vi "house_model.vi"(0 "T_out":dbl=5.0, 1 "dt":dbl=0.01, 5 "t_0":dbl, 9 "T_room_0":dbl, 14 "heat_level":dbl) -> (3 "heat_loss":dbl, 4 "T_room":dbl, 6 "error_code":dbl, 8 "t":dbl, 10 "T_heater":dbl, 15 "heat_flow":dbl)   [LabVIEW 2014]
panel:
  in  "T_heater_0":dbl
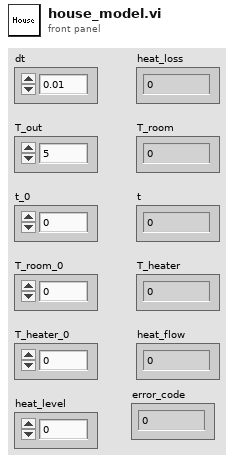
[diagram p1: front panel]
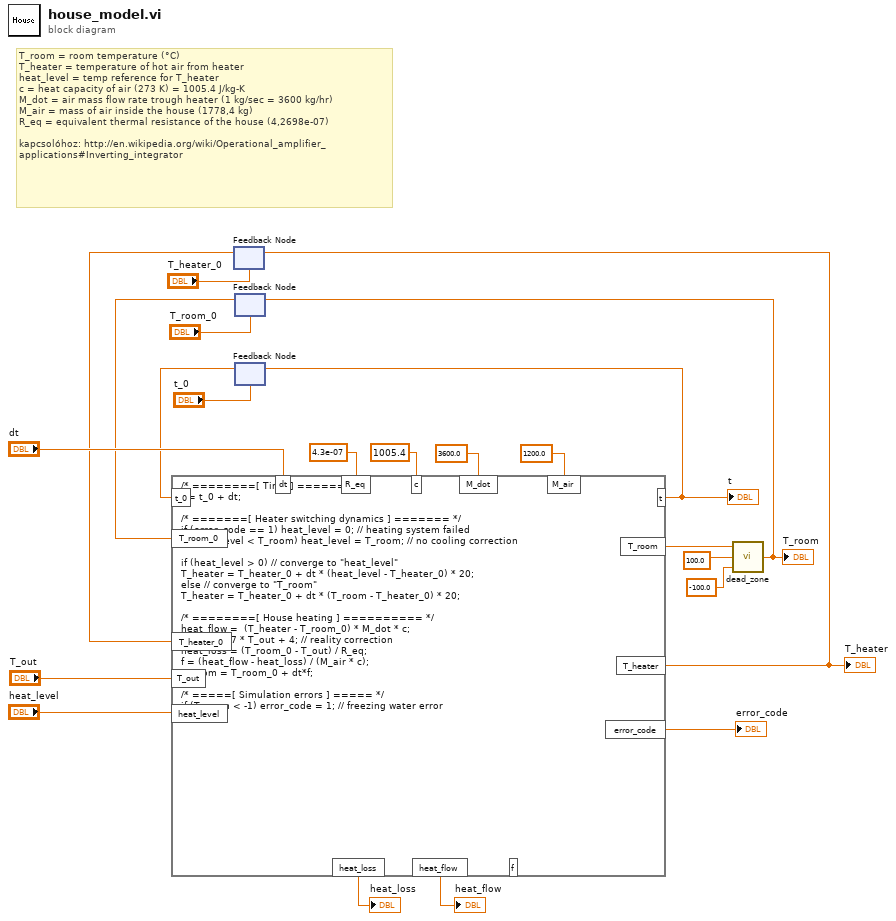
[diagram p0: block diagram]
diagram:
  # "T_room = room temperature (°C)\nT_heater = temperature of hot air from heater\nheat_level = temp reference for T_heater\nc = heat capacity of air (273 K) = 1005.4 J/kg-K\nM_dot = air mass flow rate trough heater (1 kg/sec = 3600 kg/hr)\nM_air = mass of air inside the house (1778,4 kg)\nR_eq = equivalent thermal resistance of the house (4,2698e-07)\n\nkapcsolóhoz: http://en.wikipedia.org/wiki/Operational_amplifier_applications#Inverting_integrator"
  n1 = feedback #1("T_heater_0") -> (w3:dbl)
  n2 = feedback #2("T_room_0") -> (w5:dbl)
  n3 = feedback #3("t_0") -> (w8:dbl)
  n4 = formula code="/* ========[ Time ] ======= */\nt = t_0 + dt;\n\n/* =======[ Heater switching dynamics ] ======= */\nif (error_code == 1) heat_level = 0; // heating system failed\nif (heat_level < T_room) heat_level = T_room; // no cooling correction\n\nif (heat_level > 0) // converge to \"heat_level\"\nT_heater = T_heater_0 + dt * (heat_level - T_heater_0) * 20;\nelse // converge to \"T_room\"\nT_heater = T_heater_0 + dt * (T_room - T_heater_0) * 20;\n\n/* ========[ House heating ] ========== */\nheat_flow =  (T_heater - T_room_0) * M_dot * c;\nT_out = 0.7 * T_out + 4; // reality correction\nheat_loss = (T_room_0 - T_out) / R_eq;\nf = (heat_flow - heat_loss) / (M_air * c);\nT_room = T_room_0 + dt*f;\n\n/* =====[ Simulation errors ] ===== */\nif (T_room < -1) error_code = 1; // freezing water error"("t_0"=w8, "T_room_0"=w5, "dt"="dt", "T_out"="T_out", "c"=1005.4 ("input variable"), "M_air"=1200.0 ("input variable"), "R_eq"=4.3e-07 ("input variable"), "M_dot"=3600.0 ("input variable"), "T_heater_0"=w3, "heat_level"="heat_level") -> ("t"=w7:dbl, "T_room"=w12:dbl, "heat_flow"=→"heat_flow":dbl, "heat_loss"=→"heat_loss":dbl, "T_heater"=w1:dbl, "error_code"=→"error_code":dbl)  [unwired: 1 out]
  "T_heater" <- w1
  "t" <- w7
  n5 = feedback-in #1(w1) -> ()
  n6 = feedback-in #3(w7) -> ()
  n7 = call "dead_zone.vi"("min"=-100.0, "max"=100.0, "number in"=w12) -> ("number out"=w6:dbl)
  "T_room" <- w6
  n8 = feedback-in #2(w6) -> ()
